vi "Read Server Internal UEs.vi"(8 "error in (no error)":errorcluster, 11 "SignalGeneratorService in":refnum<class "GreeterService.lvclass">) -> (0 "error out":errorcluster, 2 "Server Internal UEs":T1, 3 "SignalGeneratorService out":refnum<class "GreeterService.lvclass">)   [LabVIEW 2019, in "Generated_server.lvlib" / "GreeterService.lvclass"]
uses:
  GreeterService.lvclass
  typeDefs/Server Internal UEs.ctl
  typeDefs/Server Internal Message.ctl
  GreeterService.lvclass/GreeterService.ctl
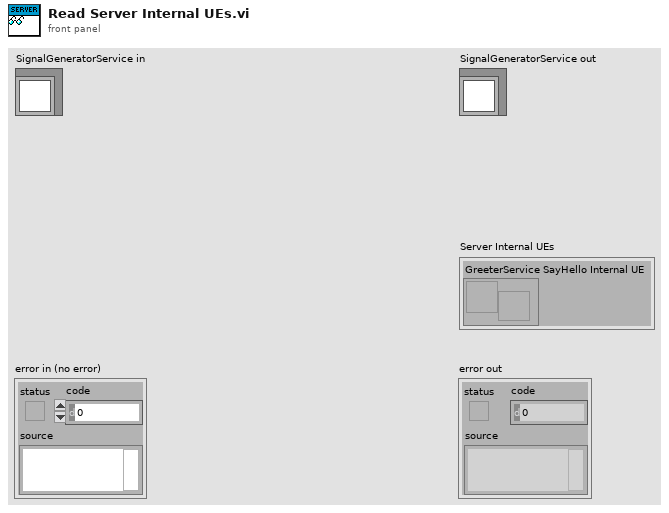
[diagram p1: front panel]
types:
  T1 = typedef "Generated_server.lvlib/GreeterService.lvclass/Server Internal UEs.ctl" = cluster{"GreeterService SayHello Internal UE":refnum<user-event>}
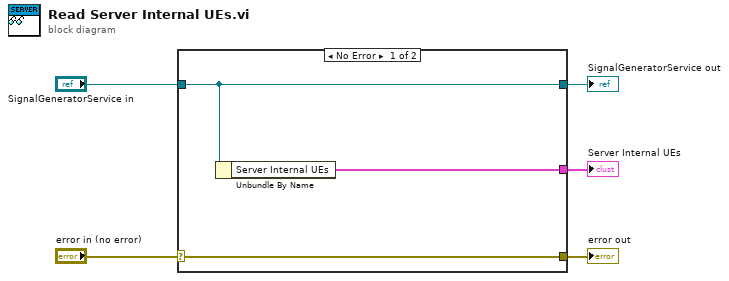
[diagram p0: block diagram]
diagram:
  n1 = case shown="No Error" "error in (no error)" {
    selector: "error in (no error)" -> [w8 w9]
    tunnel: [w8 w9] -> w4
    tunnel: [w7 w10] -> w2
    tunnel: "SignalGeneratorService in" -> [w7 w10]
    tunnel: [w6 _] -> w1
    frame No Error {
      n2 = Unbundle By Name(w7) -> ("Server Internal UEs"=w6:T1)
    }
    frame Error {
    }
  }
  "error out" <- w4
  "SignalGeneratorService out" <- w2
  "Server Internal UEs" <- w1
